vi "PAWL-LOCKS.vi"(8 "error in":errorcluster) -> (0 "error out":errorcluster, 1 "RIGHT MATCHED?":bool, 2 "LEFT MATCHED?":bool)   [LabVIEW 2020]
uses:
  Robot Global Data.vi
  <vilib>/Rock Robotics/Network Tables/NT Read Boolean.vi
  <vilib>/Rock Robotics/Network Tables/NT Write Number.vi
panel:
  out "MATCHED?":bool[](array[boolean])
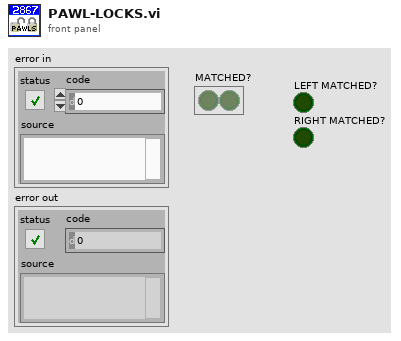
[diagram p1: front panel]
types:
  T1 = cluster{"RANGE":u16, "UNLOCKED angle":i32, "LOCKED angle":i32}
  T2 = typedef "WPI_ServoDeviceRef.ctl" = cluster{"DeviceStatus":errorcluster, "PWM Channel":T3, "DeadBand":T4}
  T3 = typedef "FPGA_DIOPWMChannel.ctl" = enum8{"PWM 0", "PWM 1", "PWM 2", "PWM 3", "PWM 4", "PWM 5", "PWM 6", "PWM 7", "PWM 8", "PWM 9", "PWM MXP 0", "PWM MXP 1", "PWM MXP 2", "PWM MXP 3", "PWM MXP 4", "PWM MXP 5", "PWM MXP 6", "PWM MXP 7", "PWM MXP 8", "PWM MXP 9", "Invalid"}
  T4 = typedef "WPI_PWMDeadband.ctl" = cluster{"Name":string, "maxPositivePwm":i32, "minPositivePwm":i32, "centerPwm":i32, "maxNegativePwm":i32, "minNegativePwm":i32, "angularRange":u16}
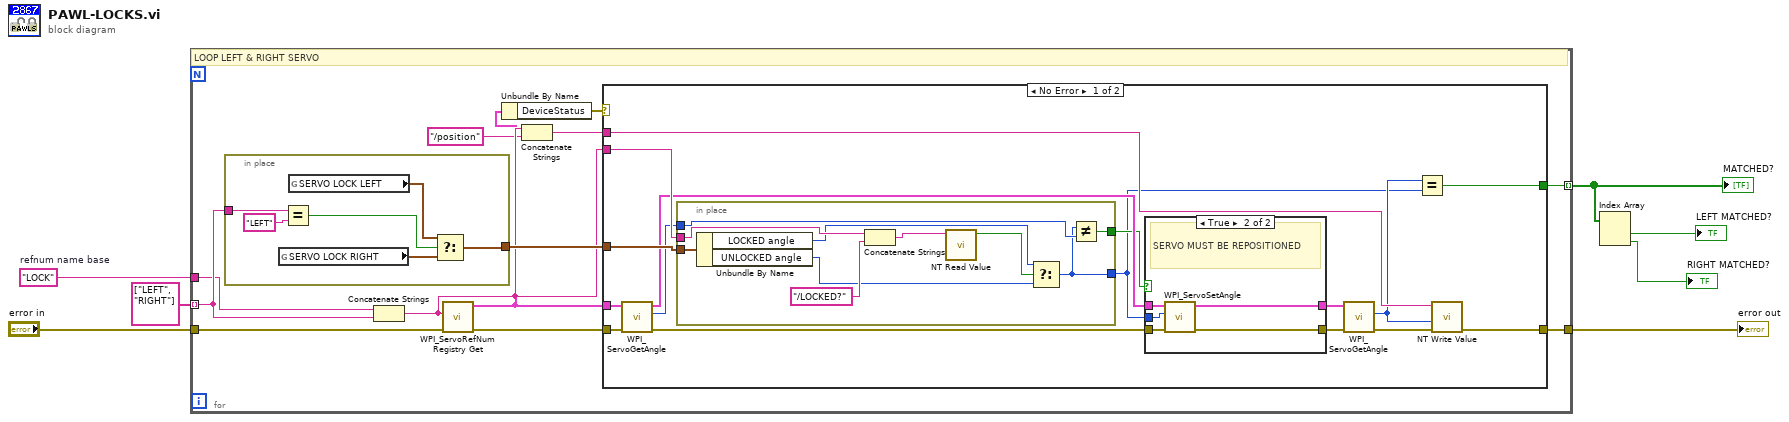
[diagram p0: block diagram]
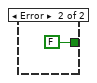
[diagram p3: hidden frame]
diagram:
  w6 = "LOCK"  # refnum name base
  n1 = for {
    tunnel: string[] ["LEFT", "RIGHT"] -> [w18] mode=indexing
    tunnel: "error in" -> [w17]
    tunnel: w6 -> [w16]
    tunnel: [w11] -> w5
    tunnel: [w10] -> w4 mode=indexing
    # "LOOP LEFT & RIGHT SERVO"
    n2 = in-place {
      in-place-border: w18 -> [w58]
      in-place-border: [w54] -> w19
      n3 = global read "Robot Global Data.vi" "SERVO LOCK RIGHT"() -> (w55:T1)
      n4 = Equal?(x=w58, y="LEFT") -> (x = y?=w59:bool)
      n5 = global read "Robot Global Data.vi" "SERVO LOCK LEFT"() -> (w56:T1)
      n6 = Select(t=w56, s=w59, f=w55) -> (s? t:f=w54:T1)
    }
    n7 = Concatenate Strings(w16, w18) -> (w15:string)
    n8 = call <vilib>:"WPI_ServoRefNum Registry Get.vi"("error in (no error)"=w17, "refnum name"=w15) -> ("error out"=w14:errorcluster, "ServoDeviceRef"=w8:T2)  [unwired: 8 in]
    n9 = Unbundle By Name(w8) -> ("DeviceStatus"=w9:errorcluster)
    n10 = Concatenate Strings(w15, "/position" ("string")) -> (w12:string)
    n11 = case shown="No Error" w9 {
      tunnel: w19 -> [w35 _]
      tunnel: w15 -> [w34 _]
      tunnel: w8 -> [w33 _]
      tunnel: w14 -> [w32 _]
      tunnel: w12 -> [w31 _]
      tunnel: [w23 _] -> w11
      tunnel: [w20 FALSE] -> w10
      frame No Error {
        n12 = call <vilib>:"WPI_ServoGetAngle.vi"("ServoDeviceRef"=w33, "error in (no error)"=w32) -> ("ServoDeviceRef"=w29:T2, "Angle"=w30:u16, "error out"=w28:errorcluster)  [unwired: 6 in]
        n13 = in-place {
          in-place-border: w35 -> [w52]
          in-place-border: w34 -> [w49]
          in-place-border: w30 -> [w45]
          in-place-border: [w44] -> w27
          in-place-border: [w43] -> w21
          n14 = Unbundle By Name(w52) -> ("LOCKED angle"=w47:i32, "UNLOCKED angle"=w46:i32)
          n15 = Concatenate Strings(w49, "/LOCKED?" ("string")) -> (w51:string)
          n16 = call-poly <vilib>:"NT Read Value.vi"("Name"=w51) -> ("Boolean"=w48:bool)  [unwired: 9 in, 1 out]
          n17 = Select(t=w47, s=w48, f=w46) -> (s? t:f=w43:i32)
          n18 = Not Equal?(x=w43, y=w45) -> (x != y?=w44:bool)
        }
        n19 = case shown="True" w27 {
          tunnel: w29 -> [w37 w42]
          tunnel: w28 -> [w36 w41]
          tunnel: w21 -> [_ w38]
          tunnel: [w37 w40] -> w26
          tunnel: [w36 w39] -> w25
          frame False {
            # "SERVO ALREADY IN POSITION"
          }
          frame True {
            # "SERVO MUST BE REPOSITIONED"
            n20 = call <vilib>:"WPI_ServoSetAngle.vi"("error in (no error)"=w41, "Angle"=w38, "ServoDeviceRef"=w42) -> ("error out"=w39:errorcluster, "ServoDeviceRef"=w40:T2)  [unwired: 7 in]
          }
        }
        n21 = call <vilib>:"WPI_ServoGetAngle.vi"("ServoDeviceRef"=w26, "error in (no error)"=w25) -> ("Angle"=w22:u16, "error out"=w24:errorcluster)  [unwired: 6 in, 1 out]
        n22 = Equal?(x=w22, y=w21) -> (x = y?=w20:bool)
        n23 = call-poly <vilib>:"NT Write Value.vi"("error in"=w24, "Numeric"=w22, "Name"=w31) -> ("error out"=w23:errorcluster)  [unwired: 8 in]
      }
      frame Error {
      }
    }
  }
  "error out" <- w5
  "MATCHED?" <- w4
  n24 = Index Array(array=w4) -> (element #1=→"LEFT MATCHED?":bool, element #2=→"RIGHT MATCHED?":bool)  [unwired: 2 in]
